vi "set_bit_depth.vi"(7 "calculate by timing? (F)":bool, 8 "error in (no error)":errorcluster, 10 "bit depth":i8, 11 "FPGAWrapperMH120124FrameScan_PXI7813R in":refnum<class "FPGAWrapperMH120124FrameScan_PXI7813R.lvclass">) -> (0 "error out":errorcluster, 3 "FPGAWrapperMH120124FrameScan_PXI7813R out":refnum<class "FPGAWrapperMH120124FrameScan_PXI7813R.lvclass">)   [LabVIEW 2010, in "FPGAWrapperMH120124FrameScan_PXI7813R.lvclass"]
uses:
  FPGAWrapperMH120124FrameScan_PXI7813R.lvclass
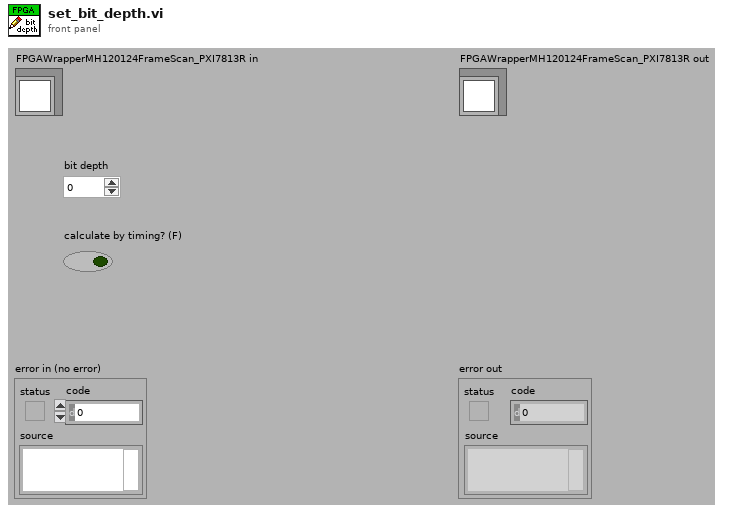
[diagram p1: front panel]
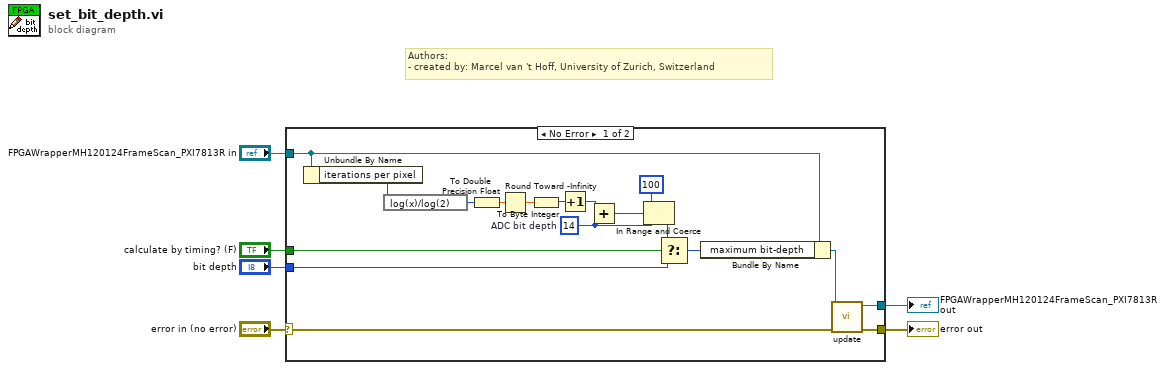
[diagram p0: block diagram]
diagram:
  # "Authors: \n- created by: Marcel van 't Hoff, University of Zurich, Switzerland"
  n1 = case shown="No Error" "error in (no error)" {
    selector: "error in (no error)" -> [w10 w26]
    tunnel: [w9 w26] -> w5
    tunnel: [w7 w25] -> w3
    tunnel: "FPGAWrapperMH120124FrameScan_PXI7813R in" -> [w16 w25]
    tunnel: "bit depth" -> [w12 _]
    tunnel: "calculate by timing? (F)" -> [w14 _]
    frame No Error {
      w22 = i8 14  # ADC bit depth
      n2 = Unbundle By Name(w16) -> ("iterations per pixel"=w15:i32)
      n3 = expression code="log(x)/log(2)"(w15) -> (w17:i32)
      n4 = To Double Precision Float(number=w17) -> (double precision float=w19:dbl)
      n5 = Round Toward -Infinity(1:w19) -> (0:w18:dbl)
      n6 = To Byte Integer(number=w18) -> (8bit integer=w20:i8)
      n7 = Increment(x=w20) -> (x+1=w21:i8)
      n8 = Add(x=w21, y=w22) -> (x+y=w23:i8)
      n9 = In Range and Coerce(upper limit=i8 100, x=w23, lower limit=w22) -> (coerced(x)=w13:i8)  [unwired: 1 out]
      n10 = Select(t=w13, s=w14, f=w12) -> (s? t:f=w11:i8)
      n11 = Bundle By Name(cluster=w16, "maximum bit-depth"=w11) -> (w8:refnum<class "FPGAWrapperMH120124FrameScan_PXI7813R.lvclass">)
      n12 = call-dynamic "update.vi"("error in (no error)"=w10, "FPGAWrapperMH120124FrameScan_PXI7813R in"=w8) -> ("error out"=w9:errorcluster, "FPGAWrapperMH120124FrameScan_PXI7813R out"=w7:refnum<class "FPGAWrapperMH120124FrameScan_PXI7813R.lvclass">)  [unwired: 8 in]
    }
    frame Error {
    }
  }
  "error out" <- w5
  "FPGAWrapperMH120124FrameScan_PXI7813R out" <- w3
